vi "Fit comparison.vi"() -> ()   [LabVIEW 2012]
uses:
  <vilib>/Analysis/6fits.llb/Curve Fitting Criteria.ctl
  <vilib>/Analysis/NI_AAL_SigProc.lvlib
  <vilib>/Analysis/NI_AALPro.lvlib
panel:
  in  "method":T1 items=["Least Square", "Least Absolute Residual", "Bisquare"]
  out "residue":dbl
  out "standard deviation":dbl
  out "amplitude":dbl
  out "Intensity vs. Pixel location":dbl[][](graph)
  out "center":dbl
  out "Locations":dbl[](array[numeric])
  out "# found":i32
  out "Amplitudes":dbl[](array[numeric])
  out "Amplitude":dbl=52.79427246119703
  out "FWHM":dbl=5.342259070694774
  out "Center":dbl=10.468826714487445
  # "manual gaussian"
  # "peak find (quad)"
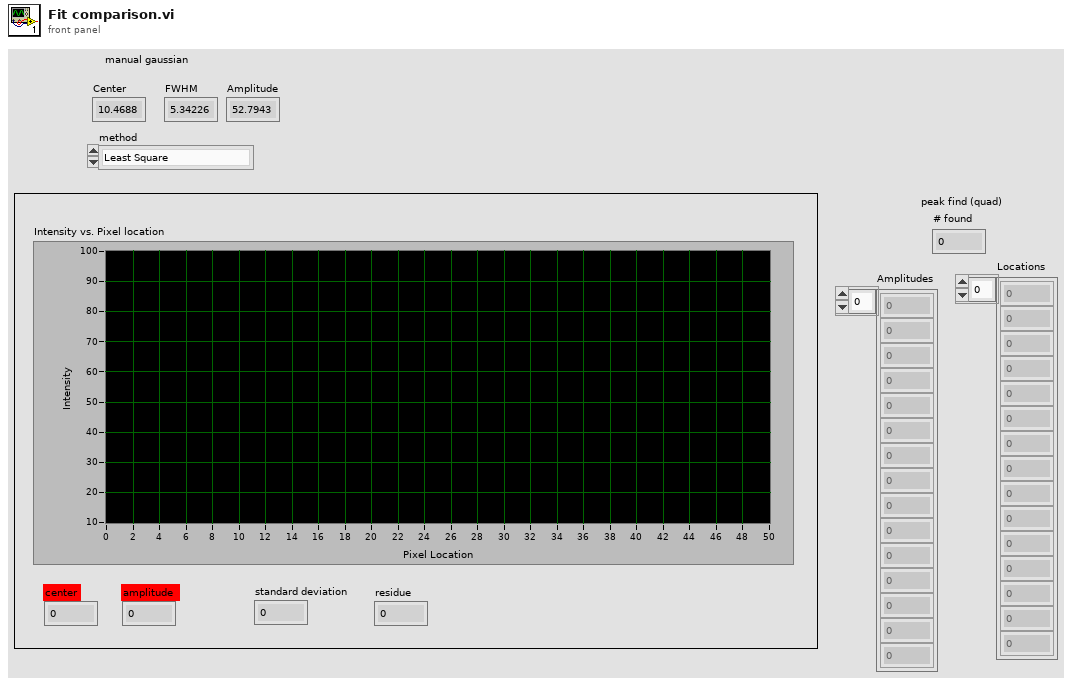
[diagram p1: front panel]
types:
  T1 = typedef "NI_AALPro.lvlib/Curve Fitting Criteria.ctl" = u16
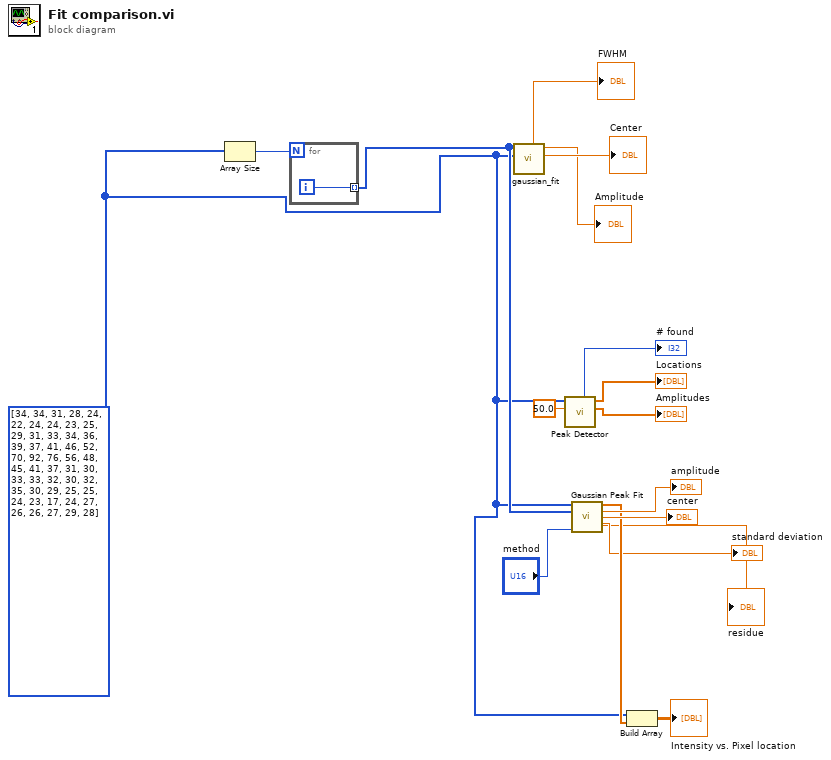
[diagram p0: block diagram]
diagram:
  w1 = i32[] [34, 34, 31, 28, 24, 22, 24, 24, 23, 25, 29, 31, 33, 34, 36, 39, 37, 41, 46, 52, 70, 92, 76, 56, 48, 45, 41, 37, 31, 30, 33, 33, 32, 30, 32, 35, 30, 29, 25, 25, 24, 23, 17, 24, 27, 26, 26, 27, 29, 28] ("subarray")
  n1 = Array Size(array=w1) -> (size(s)=w17:i32)
  n2 = for {
    N: w17 -> [_]
    tunnel: [w18] -> w6 mode=indexing
    i -> [w18]
  }
  n3 = call "gaussian_fit.vi"("Y Values"=w1, "X Values"=w6) -> ("Center"=→"Center":dbl, "Amplitude"=→"Amplitude":dbl, "FWHM"=→"FWHM":dbl)  [unwired: 2 in, 3 out]
  n4 = call <vilib>:"Peak Detector.vi"("threshold"=50.0, "X"=w1) -> ("Amplitudes"=→"Amplitudes":dbl[], "Locations"=→"Locations":dbl[], "# found"=→"# found":i32)  [unwired: 5 in, 2 out]
  n5 = call <vilib>:"Gaussian Peak Fit.vi"("Y"=w1, "X"=w6, "method"="method") -> ("Best Gaussian Fit"=w4:dbl[], "amplitude"=→"amplitude":dbl, "center"=→"center":dbl, "standard deviation"=→"standard deviation":dbl, "residue"=→"residue":dbl)  [unwired: 6 in, 2 out]
  n6 = Build Array(w1, w4) -> (→"Intensity vs. Pixel location":dbl[][])
